vi "4_transparency_plane_main.vi"() -> ()   [LabVIEW 2019]
uses:
  Shared VIs/TypeDef_TDMS_States.ctl
  <vilib>/myRIO/Common/Instrument Driver Framework/myRIO v1.0/Encoder/typedefs/Encoder Signal Mode.ctl
  Shared VIs/ModelSpecific/ETHMikeModel.ctl
  Shared VIs/ModelSpecific/ReadOnlyGlobalActions.ctl
  <vilib>/myRIO/Instrument Drivers/Onboard IO/AI/typedefs/AI Reference.ctl
  <vilib>/myRIO/Common/Instrument Driver Framework/Utilities/typedefs/myRIO Generic Hardware Reference.ctl
  <vilib>/myRIO/Common/Instrument Driver Framework/Utilities/typedefs/Hardware Version Enum.ctl
  <vilib>/myRIO/Common/Instrument Driver Framework/Utilities/typedefs/myRIO v1.0 Reference.ctl
  <vilib>/myRIO/Common/Instrument Driver Framework/Utilities/typedefs/Generic FPGA Reference.ctl
  <vilib>/myRIO/Common/Instrument Driver Framework/myRIO v1.0/AI/typedefs/AI Channels List.ctl
  <vilib>/myRIO/Common/Instrument Driver Framework/myRIO v1.0/AI/typedefs/AI Channels Enum.ctl
  <vilib>/myRIO/Common/Instrument Driver Framework/Utilities/typedefs/Analog Scaling Constants List.ctl
  <vilib>/myRIO/Common/Instrument Driver Framework/Utilities/typedefs/Analog Scaling Constants.ctl
  <vilib>/userDefined/High Color/nirio_resource_hc.ctl
  <vilib>/myRIO/Instrument Drivers/Onboard IO/AO/typedefs/AO Reference.ctl
  <vilib>/myRIO/Common/Instrument Driver Framework/myRIO v1.0/AO/typedefs/AO Channels List.ctl
  <vilib>/myRIO/Common/Instrument Driver Framework/myRIO v1.0/AO/typedefs/AO Channels Enum.ctl
  <vilib>/Platform/TimedLoop/XDataNode/timing_clust.ctl
  <vilib>/Platform/TimedLoop/XDataNode/nitl_modes.ctl
  <vilib>/Platform/TimedLoop/XDataNode/wakeup.ctl
  <vilib>/Analysis/3filter.llb/Filter Passband Type.ctl
  <vilib>/myRIO/Common/Instrument Driver Framework/myRIO v1.0/AI/vis/myRIO v1.1 Open AI.vi
  <vilib>/myRIO/Common/Instrument Driver Framework/myRIO v1.0/AO/vis/myRIO v1.1 Open AO.vi
  <vilib>/myRIO/Common/Instrument Driver Framework/Utilities/vis/Validate Channels.vi
  <vilib>/myRIO/Common/Instrument Driver Framework/myRIO v1.0/AI/vis/myRIO v1.0 Reserve AI.vi
  <vilib>/myRIO/Common/Instrument Driver Framework/myRIO v1.0/AO/vis/myRIO v1.0 Reserve AO.vi
  <vilib>/myRIO/Common/Instrument Driver Framework/myRIO v1.0/AI/vis/myRIO v1.0 Close AI.vi
  <vilib>/myRIO/Common/Instrument Driver Framework/myRIO v1.0/AO/vis/myRIO v1.0 Close AO.vi
  <vilib>/myRIO/Common/Instrument Driver Framework/myRIO v1.0/Encoder/vis/myRIO v1.0 Close Encoder.vi
  <vilib>/myRIO/Common/Instrument Driver Framework/myRIO v1.0/AI/vis/myRIO v1.0 Build MUX Configuration AI.vi
  <vilib>/myRIO/Common/Instrument Driver Framework/myRIO v1.0/Resource Manager/vis/myRIO v1.0 Reserve Channel List.vi
  <vilib>/myRIO/Common/Instrument Driver Framework/myRIO v1.0/AO/vis/myRIO v1.0 Build MUX Configuration AO.vi
  <vilib>/myRIO/Common/Instrument Driver Framework/myRIO v1.0/AI/vis/myRIO v1.0 Unreserve AI.vi
  <vilib>/myRIO/Common/Instrument Driver Framework/myRIO v1.0/AO/vis/myRIO v1.0 Unreserve AO.vi
  <vilib>/myRIO/Common/Instrument Driver Framework/myRIO v1.0/Encoder/vis/myRIO v1.0 Unreserve Encoder.vi
  <vilib>/myRIO/Common/Instrument Driver Framework/myRIO v1.0/Resource Manager/vis/myRIO v1.0 Reserve Channel.vi
  <vilib>/myRIO/Common/Instrument Driver Framework/myRIO v1.0/Resource Manager/vis/myRIO v1.0 Unreserve Channel.vi
  <vilib>/myRIO/Common/Instrument Driver Framework/myRIO v1.0/Resource Manager/vis/myRIO v1.0 Unreserve Channel List.vi
  <vilib>/myRIO/Common/Instrument Driver Framework/myRIO v1.0/Encoder/vis/myRIO v1.0 Build MUX Configuration Encoder.vi
  <vilib>/myRIO/Common/Instrument Driver Framework/myRIO v1.0/Resource Manager/vis/myRIO v1.0 Build Mutex Name.vi
  <vilib>/myRIO/Common/Instrument Driver Framework/myRIO v1.0/Resource Manager/vis/myRIO v1.0 Create Configuration List.vi
  <vilib>/Utility/VariantDataType/GetNumericInfo.vi
  <vilib>/Utility/error.llb/Error Cluster From Error Code.vi
  <vilib>/myRIO/Common/Instrument Driver Framework/myRIO v1.0/myRIO v1.1 Open.vi
  <vilib>/myRIO/Common/Instrument Driver Framework/myRIO v1.0/AO/vis/myRIO v1.0 Get Scaling Constants AO.vi
  <vilib>/myRIO/Common/Instrument Driver Framework/Utilities/vis/IO Manager.vi
  <vilib>/myRIO/Common/Instrument Driver Framework/Utilities/vis/Configuration Manager.vi
  <vilib>/myRIO/Common/Instrument Driver Framework/myRIO v1.0/myRIO v1.0 Close.vi
  <vilib>/myRIO/Common/Instrument Driver Framework/myRIO v1.0/AO/vis/myRIO v1.0 Write AO.vi
  <vilib>/myRIO/Common/Instrument Driver Framework/myRIO v1.0/AI/vis/myRIO v1.0 Get Scaling Constants AI.vi
  <vilib>/myRIO/Common/Instrument Driver Framework/myRIO v1.0/AI/vis/myRIO v1.0 Read AI.vi
  <vilib>/myRIO/Common/Instrument Driver Framework/myRIO v1.0/Encoder/vis/myRIO v1.0 Read Encoder.vi
  <vilib>/myRIO/Common/Instrument Driver Framework/myRIO v1.0/Encoder/vis/myRIO v1.0 Enable Encoder.vi
  <vilib>/myRIO/Common/Instrument Driver Framework/myRIO v1.0/Encoder/vis/myRIO v1.0 Shutdown Encoder.vi
  <vilib>/myRIO/Common/Instrument Driver Framework/myRIO v1.0/Resource Manager/vis/myRIO v1.0 Configure IO.vi
  <vilib>/myRIO/Instrument Drivers/Onboard IO/AO/vis/myRIO AO Open.xnode
  <vilib>/myRIO/Instrument Drivers/Onboard IO/AI/vis/myRIO AI Open.xnode
  <vilib>/platform/TimedLoop/XDataNode/XDataNode.xnode
  <vilib>/myRIO/Instrument Drivers/Onboard IO/AO/AO.lvlib
  <vilib>/myRIO/Instrument Drivers/Onboard IO/Encoder/Encoder.lvlib
  <vilib>/myRIO/Instrument Drivers/Onboard IO/AI/AI.lvlib
  <vilib>/Platform/TimedLoop/XDataNode/XDNodeRunTimeDep.lvlib
  <vilib>/Analysis/NI_AALBase.lvlib
  <vilib>/ptbypt/NI_PtbyPt.lvlib
panel:
  in  "TDMS Storage File Input":string
  out "TDMS States":T1
  out "Current [A]":dbl
  out "Voltage":dbl
  out "Time (ms)":dbl
  out "Velocity encoder LP [deg/s]":dbl
  out "Velocity unfiltered [deg/s]":dbl
  out "Force unfiltered [N]":dbl
  in  "Save data?":bool
  out "Force [N]":dbl
  out "Force Chart":dbl(graph)
  out "Velocity [deg/s]":dbl
  out "Velocity Chart":dbl(graph)
  out "Position [deg]":dbl
  out "Position Chart":dbl(graph)
  in  "stop":bool
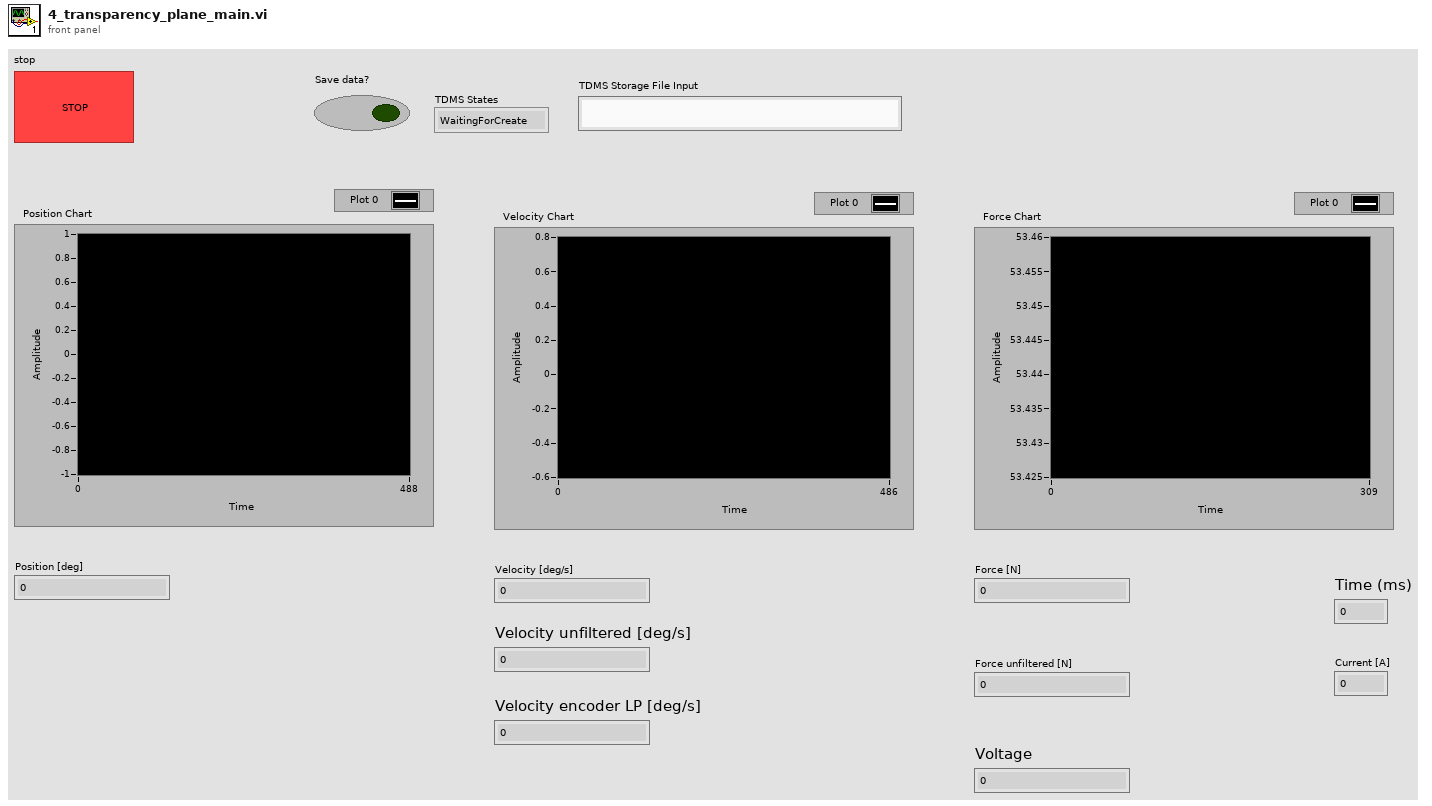
[diagram p1: front panel]
types:
  T1 = typedef "TypeDef_TDMS_States.ctl" = enum16{"WaitingForCreate", "Create", "Buffering", "Flushing", "Write", "Close"}
  T2 = typedef "nirio_resource_hc.ctl" = tag
  T3 = typedef "Hardware Version Enum.ctl" = enum16{"Unknown", "myRIO-1900", "myRIO-1950", "roboRIO", "NI ELVIS RIO CM", "ELVIS III"}
  T4 = enum16{"open", "open or create", "create or replace", "create", "open (read-only)"}
  T5 = typedef "XDNodeRunTimeDep.lvlib/timing_clust.ctl" = cluster{"Expected End [f-1]":u64, "Actual End [f-1]":u64, "Finished Late? [f-1]":bool, "Expected End [i-1]":u64, "Actual End [i-1]":u64, "Finished Late? [i-1]":bool, "Expected Start [i]":u64, "Actual Start [i]":u64, "Expected Start [f]":u64, "Actual Start [f]":u64, "Source Name":string, "Structure Name":string, "Period":i64, "Deadline":i64, "Offset":i64, "Start":i64, "Priority":i32, "Timeout":i32, "Mode":T6, "Wakeup Reason":T7, "Error":errorcluster, "Source Type":string, "Secondary Source Type":string, "Global End Time":u64, "Global Start Time":u64, "Frame Duration":u64, "Iteration Duration":u64, "Assigned CPU":i32, "I/O Scan Engine Mode":u32}
  T6 = typedef "XDNodeRunTimeDep.lvlib/nitl_modes.ctl" = enum32{"No Change", "Process missed periods, maintain original phase", "Discard missed periods, maintain original phase", "Process missed periods, ignore original phase", "Discard missed periods, ignore original phase"}
  T7 = typedef "XDNodeRunTimeDep.lvlib/wakeup.ctl" = enum32{"Normal", "Aborted", "Asynchronous wakeup", "Timing source error", "Timed loop error", "Timeout"}
  T8 = typedef "NI_AALBase.lvlib/Filter Passband Type.ctl" = enum32{"Lowpass", "Highpass", "Bandpass", "Bandstop"}
  T9 = typedef "ReadOnlyGlobalActions.ctl" = enum16{"Initialize", "Read", "Write"}
  T10 = typedef "ETHMikeModel.ctl" = enum16{"ETH Mike #1", "ETH Mike #2", "ETH Mike #3", "ETH Mike #4", "ETH MIKE #5"}
  T11 = typedef "Encoder Signal Mode.ctl" = enum16{"Quadrature phase signal", "Step and direction signal"}
  T12 = typedef "AO.lvlib/AO Reference.ctl" = cluster{"myRIO Reference":T13, "AO Channel List":T16, "AO Scaling Constant List":T18}
  T13 = typedef "myRIO Generic Hardware Reference.ctl" = cluster{"myRIO Model":T3, "myRIO Hardware Reference":T14}
  T14 = typedef "myRIO v1.0 Reference.ctl" = cluster{"Generic FPGA Reference":T15, "Allow multiple opens":bool}
  T15 = typedef "Generic FPGA Reference.ctl" = refnum<k20>
  T16 = typedef "AO Channels List.ctl" = T17[]
  T17 = typedef "AO Channels Enum.ctl" = enum16{"Not Connected", "AudioOut/Left", "AudioOut/Right", "C/AO0", "C/AO1", "A/AO0", "A/AO1", "B/AO0", "B/AO1"}
  T18 = typedef "Analog Scaling Constants List.ctl" = T19[]
  T19 = typedef "Analog Scaling Constants.ctl" = cluster{"LSB Weight (Volts)":dbl, "Offset (Volts)":dbl, "Signed?":bool}
  T20 = typedef "AI.lvlib/AI Reference.ctl" = cluster{"myRIO Reference":T13, "AI Channels List":T21, "AI Scaling Constants List":T18}
  T21 = typedef "AI Channels List.ctl" = T22[]
  T22 = typedef "AI Channels Enum.ctl" = enum16{"Not Connected", "AudioIn/Left", "AudioIn/Right", "C/AI0", "C/AI1", "A/AI0", "A/AI1", "A/AI2", "A/AI3", "A/AI4", "A/AI5", "A/AI6", "A/AI7", "B/AI0", "B/AI1", "B/AI2", "B/AI3", "B/AI4", "B/AI5", "B/AI6", "B/AI7", "AI/AI0", "AI/AI1", "AI/AI2", "AI/AI3", "A/AI0 (DIFF)", "A/AI1 (DIFF)", "A/AI2 (DIFF)", "A/AI3 (DIFF)", "B/AI0 (DIFF)", "B/AI1 (DIFF)", "B/AI2 (DIFF)", "B/AI3 (DIFF)"}
  T23 = typedef "Encoder.lvlib/Encoder Reference.ctl" = cluster{"myRIO Reference":T13, "Encoder Channels Enum":T24}
  T24 = typedef "Encoder Channels Enum.ctl" = enum16{"Not Connected", "C/ENC0", "C/ENC1", "A/ENC", "A/ENC0", "A/ENC1", "A/ENC2", "A/ENC3", "A/ENC4", "A/ENC5", "A/ENC6", "A/ENC7", "A/ENC8", "A/ENC9", "B/ENC", "B/ENC0", "B/ENC1", "B/ENC2", "B/ENC3", "B/ENC4", "B/ENC5", "B/ENC6", "B/ENC7", "B/ENC8", "B/ENC9", "DIO/ENC0", "DIO/ENC1", "DIO/ENC2", "DIO/ENC3", "DIO/ENC4"}
  T25 = typedef "TypeDefTachometerParam.ctl" = cluster{"Offset [V]":dbl, "Gain [deg/sV]":dbl}
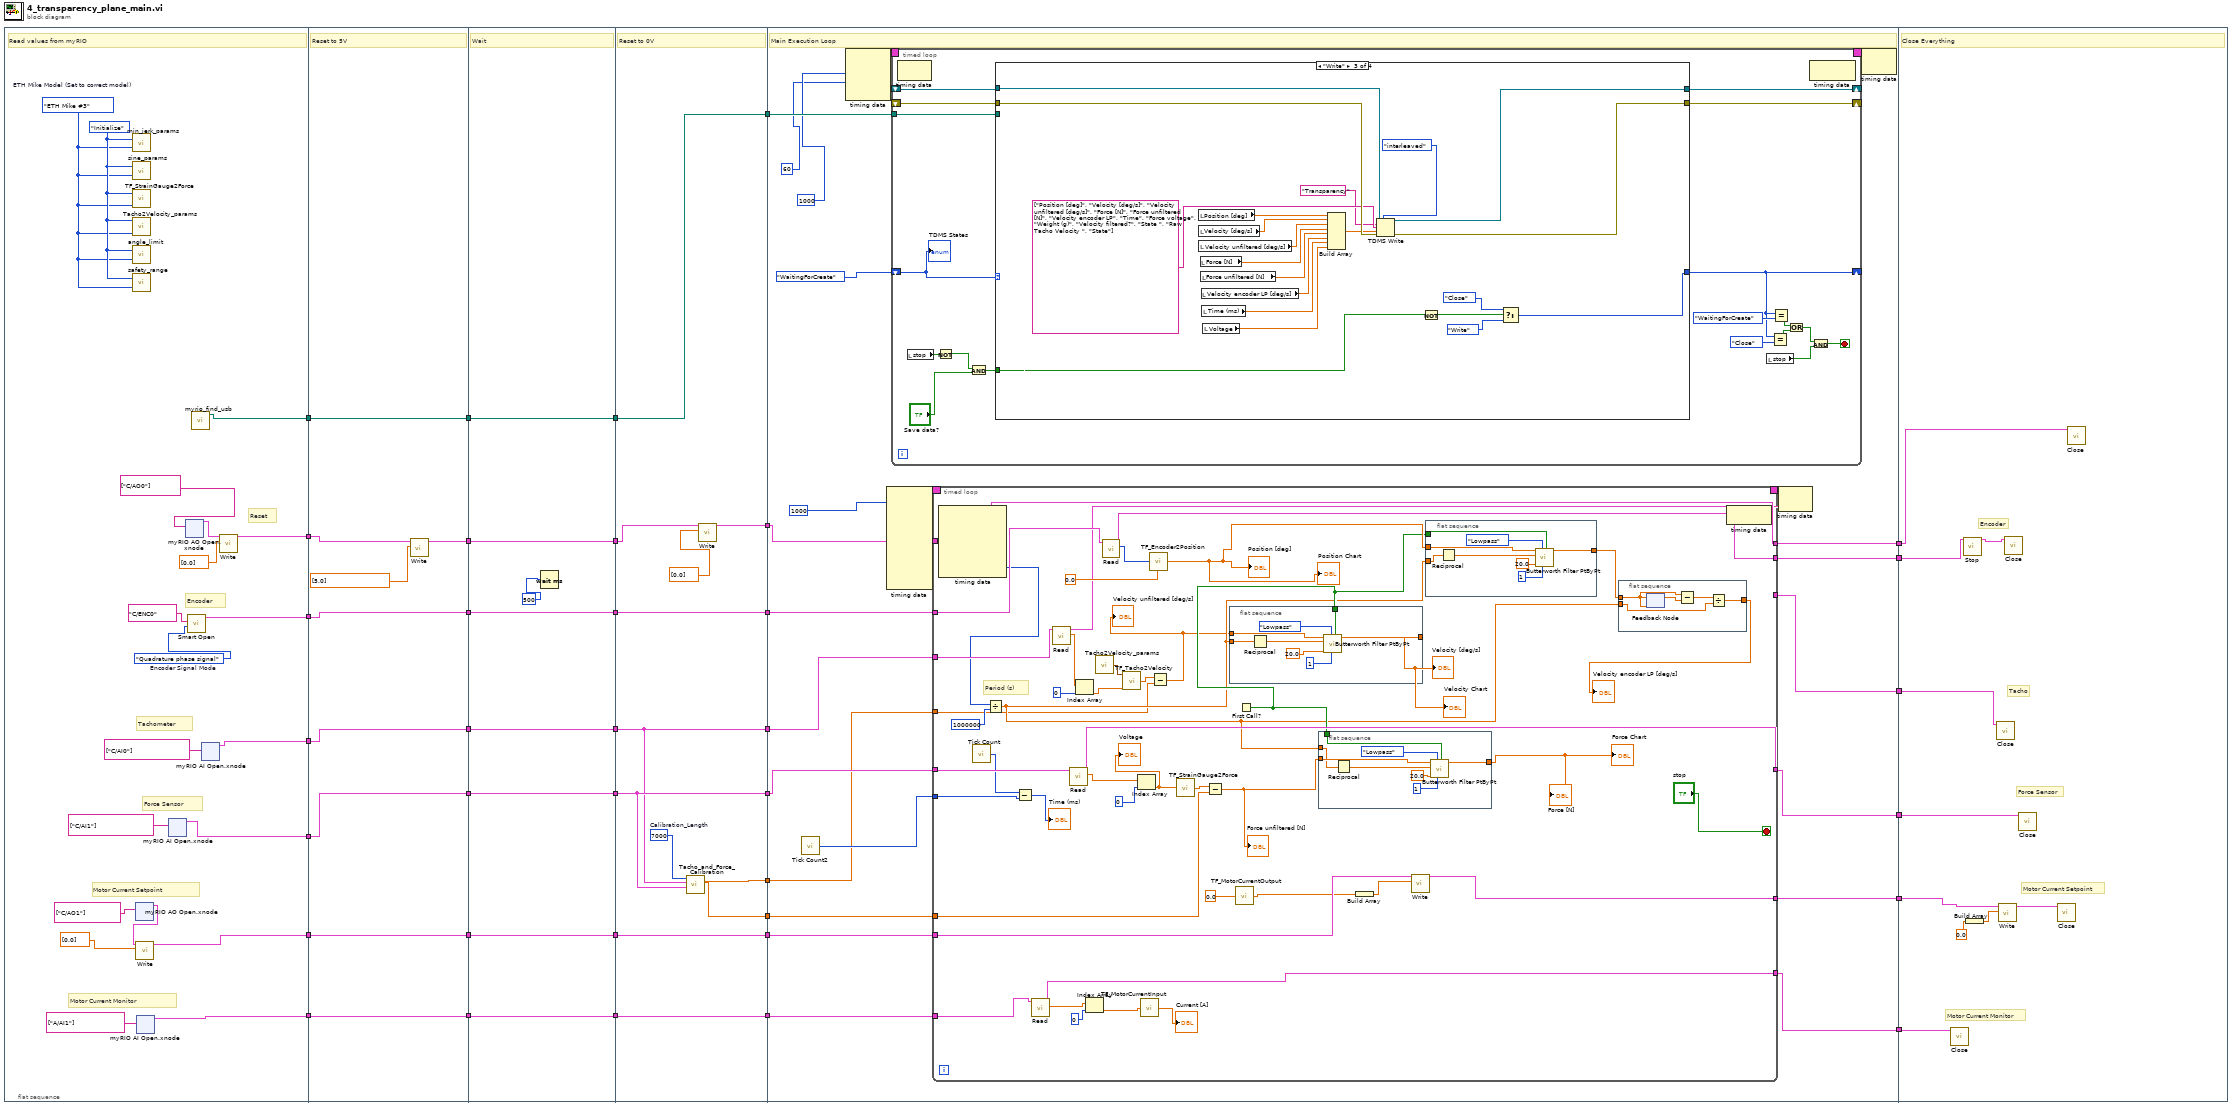
[diagram p0: block diagram]
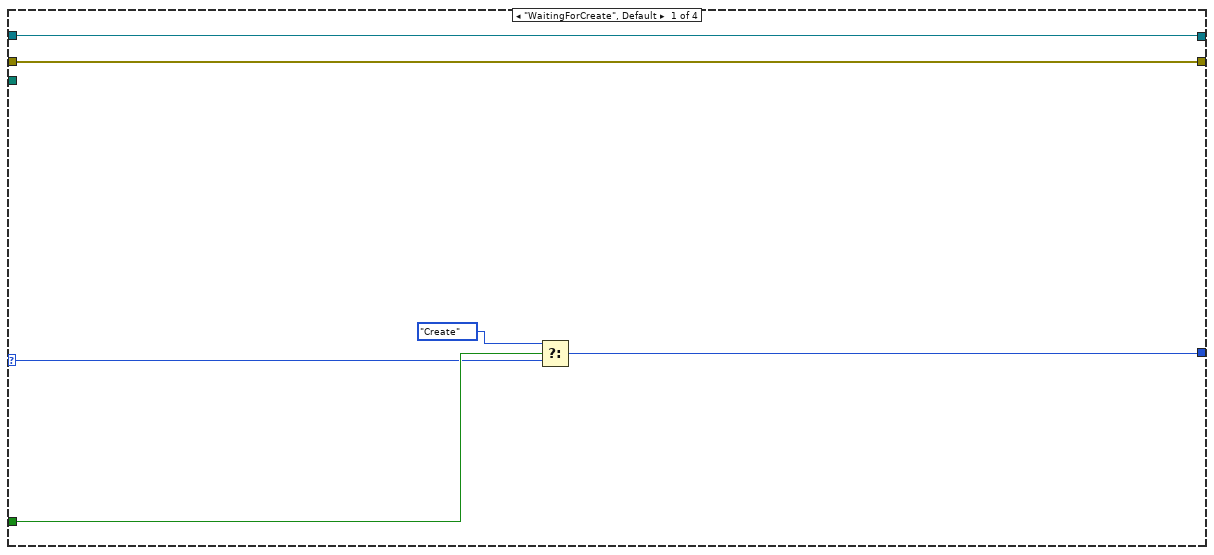
[diagram p2: hidden frame]
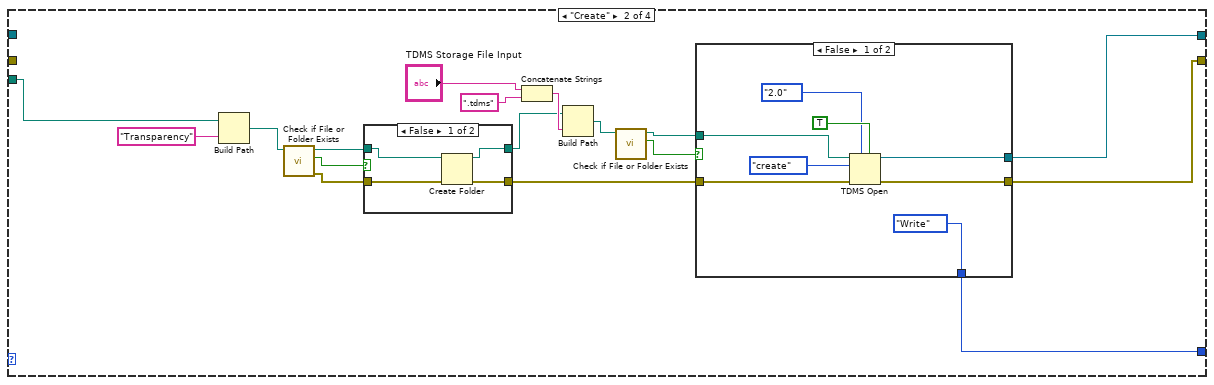
[diagram p3: hidden frame]
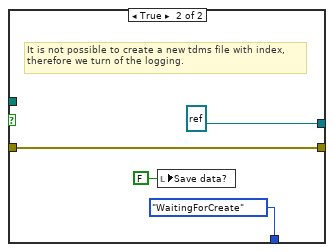
[diagram p4: hidden frame]
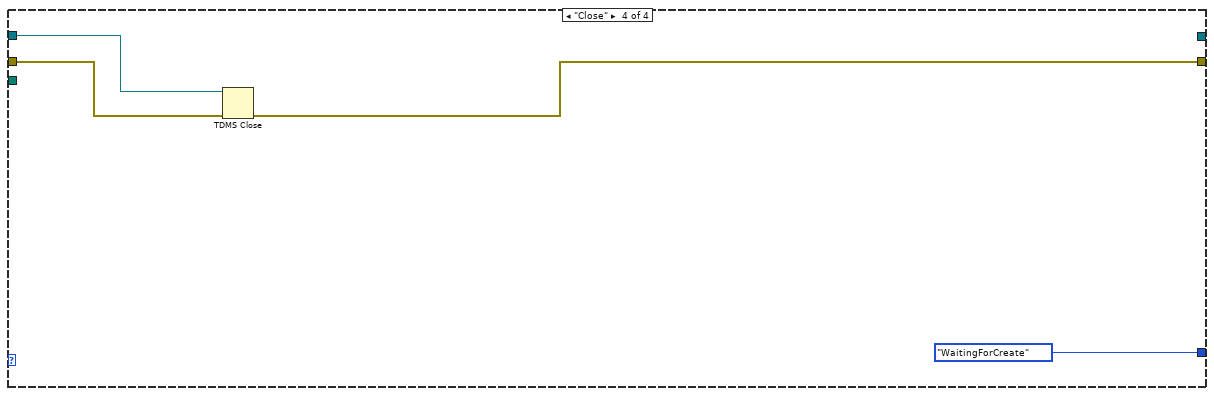
[diagram p6: hidden frame]
diagram:
  n1 = flat-sequence {
    tunnel: [w50] -> w36
    tunnel: [w49] -> w35
    tunnel: [w48] -> w34
    tunnel: [w47] -> w33
    tunnel: [w45] -> w23
    tunnel: [w41] -> w9
    tunnel: [w39] -> w4
    tunnel: w36 -> [w149]
    tunnel: w35 -> [w154]
    tunnel: w34 -> [w152]
    tunnel: w33 -> [w151]
    tunnel: [w153] -> w32
    tunnel: [w152] -> w27
    tunnel: [w151] -> w24
    tunnel: w23 -> [w150]
    tunnel: [w150] -> w20
    tunnel: [w149] -> w13
    tunnel: [w148] -> w10
    tunnel: w9 -> [w148]
    tunnel: [w147] -> w5
    tunnel: w4 -> [w147]
    tunnel: w32 -> [w162]
    tunnel: [w162] -> w31
    tunnel: [w161] -> w28
    tunnel: w27 -> [w161]
    tunnel: [w160] -> w25
    tunnel: w24 -> [w160]
    tunnel: [w159] -> w21
    tunnel: w20 -> [w159]
    tunnel: [w158] -> w14
    tunnel: w13 -> [w158]
    tunnel: [w157] -> w11
    tunnel: w10 -> [w157]
    tunnel: [w156] -> w6
    tunnel: w5 -> [w156]
    tunnel: w31 -> [w174]
    tunnel: [w173] -> w30
    tunnel: [w172] -> w29
    tunnel: w28 -> [w172]
    tunnel: [w167] -> w26
    tunnel: w25 -> [w167]
    tunnel: [w168] -> w22
    tunnel: w21 -> [w168]
    tunnel: [w171] -> w15
    tunnel: w14 -> [w171]
    tunnel: [w170] -> w12
    tunnel: w11 -> [w170]
    tunnel: [w169] -> w7
    tunnel: w6 -> [w169]
    tunnel: [w165] -> w2
    tunnel: [w164] -> w1
    tunnel: w30 -> [w196]
    tunnel: w29 -> [w194]
    tunnel: w26 -> [w192]
    tunnel: w22 -> [w191]
    tunnel: [w195] -> w19
    tunnel: [w193] -> w18
    tunnel: [w190] -> w17
    tunnel: [w189] -> w16
    tunnel: w15 -> [w186]
    tunnel: w12 -> [w181]
    tunnel: [w180] -> w8
    tunnel: w7 -> [w179]
    tunnel: [w178] -> w3
    tunnel: w2 -> [w177]
    tunnel: w1 -> [w176]
    tunnel: w19 -> [w382]
    tunnel: w18 -> [w380]
    tunnel: w17 -> [w379]
    tunnel: w16 -> [w378]
    tunnel: w8 -> [w374]
    tunnel: w3 -> [w373]
    frame #0 {
      w38 = ReadOnlyGlobalActions."Initialize" ("Action (Read)")
      w37 = ETHMikeModel."ETH Mike #3"  # ETH Mike Model (Set to correct model)
      w52 = Encoder_Signal_Mode."Quadrature phase signal"  # Encoder Signal Mode
      # "Motor Current Monitor"
      # "Motor Current Setpoint"
      # "Force Sensor"
      # "Tachometer"
      # "Encoder"
      # "Reset"
      # "Read values from myRIO"
      n2 = call "min_jerk_params.vi"("Action (Read)"=w38, "ETH Mike Model"=w37) -> ()  [unwired: 17 in, 1 out]
      n3 = call "sine_params.vi"("Action (Read)"=w38, "ETH Mike Model"=w37) -> ()  [unwired: 17 in, 1 out]
      n4 = call "TF_StrainGauge2Force.vi"("Action (Read)"=w38, "ETH Mike Model"=w37) -> ()  [unwired: 3 in, 1 out]
      n5 = call "Tacho2Velocity_params.vi"("Action (Read)"=w38, "ETH Mike Model"=w37) -> ()  [unwired: 3 in, 1 out]
      n6 = call "angle_limit.vi"("ETH Mike Model"=w37, "Action (Read)"=w38) -> ()  [unwired: 1 out]
      n7 = call "safety_range.vi"("ETH Mike Model"=w37, "Action (Read)"=w38) -> ()  [unwired: 1 out]
      n8 = xnode "myRIO AO Open.xnode"("Channel Names"=tag[] ["C/AO1"]) -> ("AO Ref Out"=w43:T12)  [unwired: 2 in, 1 out]
      n9 = call <vilib>:"Write.vi"("Values"=dbl[] [0.0], "AO Ref In"=w43) -> ("AO Ref Out"=w41:T12)  [unwired: 7 in, 1 out]
      n10 = xnode "myRIO AI Open.xnode"("Channel Names"=tag[] ["A/AI1"]) -> ("AI Ref Out"=w39:T20)  [unwired: 2 in, 1 out]
      n11 = xnode "myRIO AI Open.xnode"("Channel Names"=tag[] ["C/AI1"]) -> ("AI Ref Out"=w45:T20)  [unwired: 2 in, 1 out]
      n12 = xnode "myRIO AO Open.xnode"("Channel Names"=tag[] ["C/AO0"]) -> ("AO Ref Out"=w55:T12)  [unwired: 2 in, 1 out]
      n13 = call <vilib>:"Smart Open.vi"("Encoder Signal Mode"=w52, "Channel Name"=tag "C/ENC0") -> ("Encoder Ref Out"=w48:T23)  [unwired: 8 in, 1 out]
      n14 = call "myrio_find_usb.vi"() -> ("Largest USB Partition Path"=w50:path)  [unwired: 9 in, 2 out]
      n15 = xnode "myRIO AI Open.xnode"("Channel Names"=tag[] ["C/AI0"]) -> ("AI Ref Out"=w47:T20)  [unwired: 2 in, 1 out]
      n16 = call <vilib>:"Write.vi"("Values"=dbl[] [0.0], "AO Ref In"=w55) -> ("AO Ref Out"=w49:T12)  [unwired: 7 in, 1 out]
    }
    frame #1 {
      # "Reset to 5V"
      n17 = call <vilib>:"Write.vi"("Values"=dbl[] [5.0], "AO Ref In"=w154) -> ("AO Ref Out"=w153:T12)  [unwired: 7 in, 1 out]
    }
    frame #2 {
      # "Wait"
      n18 = Wait (ms)(milliseconds to wait=500) -> ()  [unwired: 1 out]
    }
    frame #3 {
      w166 = 7000  # Calibration_Length
      # "Reset to 0V"
      n19 = call "Tacho_and_Force_Calibration.vi"("Force Ref In"=w168, "Tacho Ref In"=w167, "Calibration_Length"=w166) -> ("Force_calib_value"=w165:dbl, "Velocity_calib_value"=w164:dbl)  [unwired: 7 in]
      n20 = call <vilib>:"Write.vi"("Values"=dbl[] [0.0], "AO Ref In"=w174) -> ("AO Ref Out"=w173:T12)  [unwired: 7 in, 1 out]
    }
    frame #4 {
      # "Main Execution Loop"
      n21 = call "Tick Count2"() -> ("Tick Count(mSec)"=w182:u32)
      n22 = node-c288(i64 1000 ("Period"), 60) -> (w188:T5)  [unwired: 2 in]
      n23 = node-c288(i64 1000 ("Period")) -> (w199:T5)  [unwired: 9 in]
      n24 = timed-loop {
        timing: w188 -> [_]
        timing-out: [_] -> w187
        shift-right: [w217] -> _
        shift-left: _ -> [w215]
        shift-right: [w216] -> _
        shift-left: _ -> [w214]
        tunnel: w186 -> [w213]
        shift-right: [w204] -> _
        shift-left: TypeDef_TDMS_States."WaitingForCreate" ("TDMS States") -> [w212]
        stop <- w200 stop-if-true
        n25 = node-c288() -> ()  [unwired: 1 in, 1 out]
        n26 = local read "stop"() -> (w209:bool)
        n27 = Not(x=w209) -> (.not. x?=w208:bool)
        n28 = And(x=w208, y="Save data?") -> (x .and. y?=w211:bool)
        n29 = case shown="\"Write\"" w212 {
          selector: w212 -> [w221 _ _ _]
          tunnel: w211 -> [w222 _ w262 _]
          tunnel: [w219 w227 w267 w281] -> w216
          tunnel: [w218 w226 w266 _] -> w217
          tunnel: w215 -> [w218 _ w260 w283]
          tunnel: w214 -> [w219 _ w271 w282]
          tunnel: w213 -> [_ w239 _ _]
          tunnel: [w220 w225 w261 TypeDef_TDMS_States."WaitingForCreate" ("TDMS States")] -> w204
          frame "WaitingForCreate", Default {
            n30 = Select(t=TypeDef_TDMS_States."Create" ("TDMS States"), s=w222, f=w221) -> (s? t:f=w220:T1)
          }
          frame "Create" {
            n31 = Build Path(base path=w239, name or relative path="Transparency") -> (appended path=w238:path)
            n32 = call <vilib>:"Check if File or Folder Exists.vi"("path"=w238) -> ("error out"=w235:errorcluster, "file or folder exists?"=w236:bool, "dup path"=w237:path)  [unwired: 8 in]
            n33 = case shown="False" w236 {
              tunnel: w237 -> [w256 w257]
              tunnel: [w255 w258] -> w228
              tunnel: w235 -> [w254 w258]
              tunnel: [w253 w257] -> w231
              frame False {
                n34 = Create Folder(path (use dialog)=w256, error in=w254) -> (created path=w253:path, error out=w255:errorcluster)  [unwired: 1 in, 1 out]
              }
              frame True {
              }
            }
            n35 = Concatenate Strings("TDMS Storage File Input", ".tdms") -> (w232:string)
            n36 = Build Path(base path=w231, name or relative path=w232) -> (appended path=w230:path)
            n37 = call <vilib>:"Check if File or Folder Exists.vi"("path"=w230) -> ("file or folder exists?"=w229:bool, "dup path"=w224:path)  [unwired: 8 in, 1 out]
            n38 = case shown="False" w229 {
              tunnel: w228 -> [w248 w252]
              tunnel: [w242 w252] -> w227
              tunnel: [w243 refnum<k34> refnum ("tdms file out")] -> w226
              tunnel: [TypeDef_TDMS_States."Write" ("TDMS States") TypeDef_TDMS_States."WaitingForCreate" ("TDMS States")] -> w225
              tunnel: w224 -> [w246 _]
              frame False {
                n39 = TDMS Open(5:TRUE, 7:enum16{"1.0", "2.0"}."2.0" ("file format version (2.0)"), 8:w248, 10:T4."create" ("operation (0:open)"), 11:w246) -> (0:w242:errorcluster, 3:w243:refnum<k34>)  [unwired: 2 in]
              }
              frame True {
                # "It is not possible to create a new tdms file with index,\ntherefore we turn of the logging."
                n40 = local write "Save data?"(FALSE ("Save data?")) -> ()
              }
            }
          }
          frame "Write" {
            n41 = local read "Position [deg]"() -> (w272:dbl)
            n42 = local read "Velocity [deg/s]"() -> (w273:dbl)
            n43 = local read "Velocity unfiltered [deg/s]"() -> (w274:dbl)
            n44 = local read "Force [N]"() -> (w275:dbl)
            n45 = local read "Force unfiltered [N]"() -> (w276:dbl)
            n46 = local read "Velocity encoder LP [deg/s]"() -> (w277:dbl)
            n47 = local read "Time (ms)"() -> (w278:dbl)
            n48 = local read "Voltage"() -> (w279:dbl)
            n49 = Build Array(w272, w273, w274, w275, w276, w277, w278, w279) -> (w270:dbl[])
            n50 = TDMS Write(0:w260, 1:enum16{"decimated", "interleaved"}."interleaved" ("data layout (0:decimated)"), 5:"Transparency" ("group name in (Untitled)"), 7:string[] ["Position [deg]", "Velocity [deg/s]", "Velocity unfiltered [deg/s]", "Force [N]", "Force unfiltered [N]", "Velocity encoder LP", "Time", "Force voltage", "Weight (g)", "Velocity filtered?", "State ", "Raw Tacho Velocity ", "State"], 9:w270, 11:w271) -> (4:w266:refnum<k34>, 15:w267:errorcluster)  [unwired: 2 out]
            n51 = Not(x=w262) -> (.not. x?=w265:bool)
            n52 = Select(t=TypeDef_TDMS_States."Close" ("TDMS States"), s=w265, f=TypeDef_TDMS_States."Write" ("TDMS States")) -> (s? t:f=w261:T1)
          }
          frame "Close" {
            n53 = TDMS Close(8:w282, 11:w283) -> (0:w281:errorcluster)  [unwired: 1 out]
          }
        }
        n54 = local read "stop"() -> (w201:bool)
        n55 = Equal?(x=w204, y=TypeDef_TDMS_States."Close" ("TDMS States")) -> (x = y?=w205:bool)
        n56 = Equal?(x=w204, y=TypeDef_TDMS_States."WaitingForCreate" ("TDMS States")) -> (x = y?=w206:bool)
        n57 = Or(x=w206, y=w205) -> (x .or. y?=w202:bool)
        n58 = node-c288() -> ()  [unwired: 1 in, 1 out]
        n59 = And(x=w202, y=w201) -> (x .and. y?=w200:bool)
        "TDMS States" <- w212
      }
      n60 = timed-loop {
        timing: w199 -> [_]
        timing-out: [_] -> w198
        tunnel: [w334] -> w195
        tunnel: w196 -> [w334]
        tunnel: w194 -> [w332]
        tunnel: [w331] -> w193
        tunnel: w192 -> [w330]
        tunnel: [w329] -> w189
        tunnel: w191 -> [w314]
        tunnel: [w322] -> w190
        tunnel: w182 -> [w311]
        tunnel: w181 -> [w308]
        tunnel: [w306] -> w180
        tunnel: w179 -> [w302]
        tunnel: [w301] -> w178
        tunnel: w177 -> [w295]
        tunnel: w176 -> [w292]
        stop <- "stop" stop-if-true
        # "Period (s)"
        n61 = node-c288() -> (w325:i64)  [unwired: 1 in, 6 out]
        n62 = call "Tick Count"() -> ("Tick Count(mSec)"=w312:u32)
        n63 = Divide(x=w325, y=1000000) -> (x/y=w317:dbl)
        n64 = Subtract(x=w312, y=w311) -> (x-y=→"Time (ms)":u32)
        n65 = call <vilib>:"Read.vi"("AI Ref In"=w302) -> ("Values"=w304:dbl[], "AI Ref Out"=w301:T20)  [unwired: 8 in, 1 out]
        n66 = call <vilib>:"Read.vi"("AI Ref In"=w330) -> ("Values"=w328:dbl[], "AI Ref Out"=w329:T20)  [unwired: 8 in, 1 out]
        n67 = call <vilib>:"Read.vi"("AI Ref In"=w314) -> ("Values"=w321:dbl[], "AI Ref Out"=w322:T20)  [unwired: 8 in, 1 out]
        n68 = Index Array(array=w328, index=0) -> (element=w299:dbl)
        n69 = Index Array(array=w304, index=0) -> (element=w303:dbl)
        n70 = call "Tacho2Velocity_params.vi"() -> ("Cluster"=w298:T25)  [unwired: 5 in]
        n71 = call <vilib>:"Read.vi"("Encoder Ref In"=w332) -> ("Counter Value"=w336:i32, "Encoder Ref Out"=w331:T23)  [unwired: 6 in, 3 out]
        n72 = call "TF_Tacho2Velocity.vi"("Tachometer Voltage [V]"=w299, "Tachometer param"=w298) -> ("Tachometer Velocity [deg/s]"=w293:dbl)  [unwired: 2 in]
        n73 = Index Array(array=w321, index=0) -> (element=w297:dbl)
        "Voltage" <- w297
        n74 = call "TF_MotorCurrentInput.vi"("Motor Current Monitor Value [V]"=w303) -> ("Current [A]"=→"Current [A]":dbl)
        n75 = call "TF_Encoder2Position.vi"("Counter Value"=w336, "Offset"=0.0) -> ("Position [deg]"=w319:dbl)  [unwired: 3 in]
        "Position Chart" <- w319
        "Position [deg]" <- w319
        n76 = Subtract(x=w293, y=w292) -> (x-y=w291:dbl)
        "Velocity unfiltered [deg/s]" <- w291
        n77 = call "TF_StrainGauge2Force.vi"("Strain Gauge Value [V]"=w297) -> ("Force [N]"=w296:dbl)  [unwired: 4 in]
        n78 = Subtract(x=w296, y=w295) -> (x-y=w294:dbl)
        "Force unfiltered [N]" <- w294
        n79 = flat-sequence {
          tunnel: w291 -> [w365]
          tunnel: w317 -> [w363]
          tunnel: [w360] -> w324
          tunnel: w318 -> [w358]
          frame #0 {
            n80 = Reciprocal(x=w363) -> (1/x=w364:dbl)
            n81 = call <vilib>:"Butterworth Filter PtByPt.vi"("initialize"=w358, "order"=1, "filter type"=Filter_Passband_Type."Lowpass", "low cutoff freq: fl"=20.0, "sampling freq: fs"=w364, "x"=w365) -> ("Filtered x"=w360:dbl)  [unwired: 3 in, 1 out]
          }
        }
        n82 = call "TF_MotorCurrentOutput.vi"("Motor Current Setpoint [A]"=0.0) -> ("Motor Current Setpoint [V]"=w307:dbl)
        n83 = First Call?() -> (First Call?: T/F=w318:bool)
        n84 = flat-sequence {
          tunnel: w294 -> [w357]
          tunnel: [w352] -> w320
          tunnel: w317 -> [w351]
          tunnel: w318 -> [w350]
          frame #0 {
            n85 = Reciprocal(x=w351) -> (1/x=w356:dbl)
            n86 = call <vilib>:"Butterworth Filter PtByPt.vi"("initialize"=w350, "order"=1, "filter type"=Filter_Passband_Type."Lowpass", "low cutoff freq: fl"=20.0, "sampling freq: fs"=w356, "x"=w357) -> ("Filtered x"=w352:dbl)  [unwired: 3 in, 1 out]
          }
        }
        n87 = Build Array(w307) -> (w309:dbl[])
        n88 = call <vilib>:"Write.vi"("Values"=w309, "AO Ref In"=w308) -> ("AO Ref Out"=w306:T12)  [unwired: 7 in, 1 out]
        n89 = flat-sequence {
          tunnel: w319 -> [w344]
          tunnel: w318 -> [w340]
          tunnel: [w338] -> w316
          tunnel: w317 -> [w337]
          frame #0 {
            n90 = Reciprocal(x=w337) -> (1/x=w343:dbl)
            n91 = call <vilib>:"Butterworth Filter PtByPt.vi"("initialize"=w340, "order"=1, "filter type"=Filter_Passband_Type."Lowpass", "low cutoff freq: fl"=20.0, "sampling freq: fs"=w343, "x"=w344) -> ("Filtered x"=w338:dbl)  [unwired: 3 in, 1 out]
          }
        }
        n92 = flat-sequence {
          tunnel: [w347] -> w315
          tunnel: w316 -> [w346]
          tunnel: w317 -> [w345]
          frame #0 {
            n93 = feedback #1(w346) -> (w349:dbl)
            n94 = feedback-in #1(w346) -> ()
            n95 = Subtract(x=w346, y=w349) -> (x-y=w348:dbl)
            n96 = Divide(x=w348, y=w345) -> (x/y=w347:dbl)
          }
        }
        n97 = node-c288() -> ()  [unwired: 1 in, 1 out]
        "Velocity Chart" <- w324
        "Velocity [deg/s]" <- w324
        "Force Chart" <- w320
        "Force [N]" <- w320
        "Velocity encoder LP [deg/s]" <- w315
      }
      n98 = node-c288(w198) -> ()  [unwired: 1 out]
      n99 = node-c288(w187) -> ()  [unwired: 1 out]
    }
    frame #5 {
      # "Motor Current Monitor"
      # "Motor Current Setpoint"
      # "Force Sensor"
      # "Tacho"
      # "Encoder"
      # "Close Everything"
      n100 = call <vilib>:"Close.vi"("AI Ref In"=w373) -> ()  [unwired: 10 in, 1 out]
      n101 = call <vilib>:"Stop.vi"("Encoder Ref In"=w380) -> ("Encoder Ref Out"=w381:T23)  [unwired: 9 in, 1 out]
      n102 = Build Array(0.0) -> (w375:dbl[])
      n103 = call <vilib>:"Close.vi"("AI Ref In"=w378) -> ()  [unwired: 10 in, 1 out]
      n104 = call <vilib>:"Write.vi"("Values"=w375, "AO Ref In"=w374) -> ("AO Ref Out"=w377:T12)  [unwired: 7 in, 1 out]
      n105 = call <vilib>:"Close.vi"("Encoder Ref In"=w381) -> ()  [unwired: 10 in, 1 out]
      n106 = call <vilib>:"Close.vi"("AI Ref In"=w379) -> ()  [unwired: 10 in, 1 out]
      n107 = call <vilib>:"Close.vi"("AO Ref In"=w377) -> ()  [unwired: 10 in, 1 out]
      n108 = call <vilib>:"Close.vi"("AO Ref In"=w382) -> ()  [unwired: 10 in, 1 out]
    }
  }
